vi "Create Host String.vi"(11 "HTTP Session in":refnum<class "Session.lvclass">) -> (2 "Host String":string, 3 "HTTP Session out":refnum<class "Session.lvclass">)   [LabVIEW 2015, in "NI_Azure_Core.lvlib" / "Session.lvclass"]
uses:
  Session.lvclass
  Format Request Parameters Mode.ctl
  Session.lvclass/Session.ctl
  Read URL Suffix.vi
  Read URL Prefix.vi
  Read Request Parameters.vi
  Read _ServiceName.vi
  Read Storage Account Name.vi
  NI_Azure_Core.lvlib
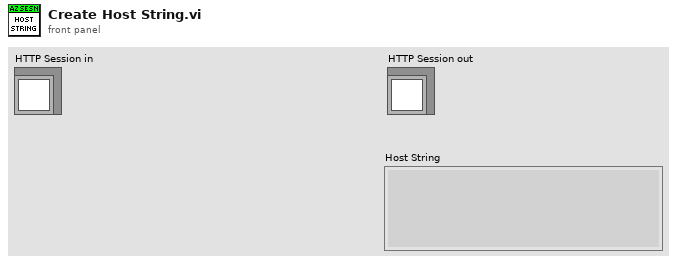
[diagram p1: front panel]
types:
  T1 = typedef "NI_Azure_Core.lvlib/Format Request Parameters Mode.ctl" = enum16{"URL", "Signing"}
  T2 = typedef "NI_Azure_Core.lvlib/Name Value Pair.ctl" = cluster{"name":string, "value":string}
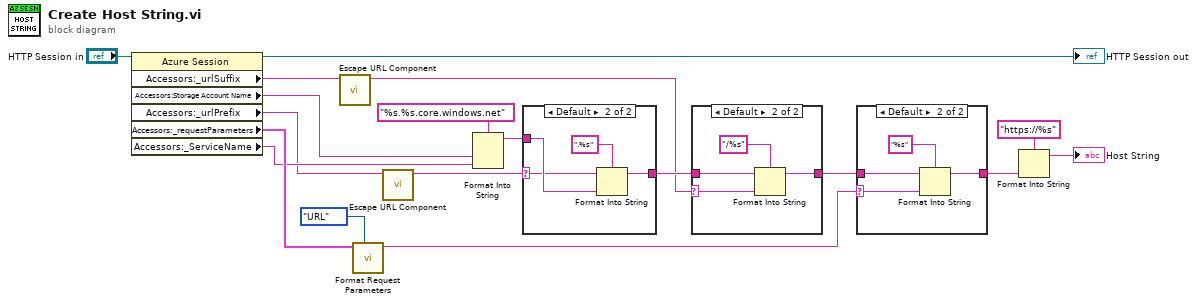
[diagram p0: block diagram]
diagram:
  n1 = property class="Azure Session"(reference="HTTP Session in") -> (reference out=→"HTTP Session out":refnum<class "Session.lvclass">, "Accessors:_urlSuffix"=w4:string, "Accessors:Storage Account Name"=w12:string, "Accessors:_urlPrefix"=w2:string, "Accessors:_requestParameters"=w11:T2[], "Accessors:_ServiceName"=w5:string)  [unwired: 1 in, 1 out]
  n2 = call "Escape URL Component.vi"("URL component in"=w4) -> ("URL component out"=w3:string)  [unwired: 10 in]
  n3 = call "Format Request Parameters.vi"("Mode"=Format_Request_Parameters_Mode."URL", "Request parameters"=w11) -> ("Parameter string"=w10:string)  [unwired: 9 in]
  n4 = call "Escape URL Component.vi"("URL component in"=w2) -> ("URL component out"=w1:string)  [unwired: 10 in]
  n5 = Format Into String(format string="%s.%s.core.windows.net" ("string"), w12, w5) -> (resulting string=w17:string)  [unwired: 2 in, 1 out]
  n6 = case shown="Default" w1 {
    selector: w1 -> [_ w20]
    tunnel: [w19 w22] -> w14
    tunnel: w17 -> [w19 w21]
    frame "" {
    }
    frame Default {
      n7 = Format Into String(format string=".%s", initial string=w20, w21) -> (resulting string=w22:string)  [unwired: 1 in, 1 out]
    }
  }
  n8 = case shown="Default" w3 {
    selector: w3 -> [_ w26]
    tunnel: [w24 w27] -> w13
    tunnel: w14 -> [w24 w25]
    frame "" {
    }
    frame Default {
      n9 = Format Into String(format string="/%s", initial string=w25, w26) -> (resulting string=w27:string)  [unwired: 1 in, 1 out]
    }
  }
  n10 = case shown="Default" w10 {
    selector: w10 -> [_ w31]
    tunnel: [w29 w32] -> w6
    tunnel: w13 -> [w29 w30]
    frame "" {
    }
    frame Default {
      n11 = Format Into String(format string="%s", initial string=w30, w31) -> (resulting string=w32:string)  [unwired: 1 in, 1 out]
    }
  }
  n12 = Format Into String(format string="https://%s" ("string"), w6) -> (resulting string=→"Host String":string)  [unwired: 2 in, 1 out]
